vi "twoMPUsI2C.vi"() -> ()   [LabVIEW 2016]
uses:
  <vilib>/MakerHub/LINX/LMH-LINX.lvlib
  <vilib>/MakerHub/LINX/Public/Sensors/Accelerometer/MPU60X0/MPU60X0.lvlib
  <vilib>/MakerHub/LINX/Public/Sensors/Accelerometer/MPU60X0/AccelFullScaleRanges.ctl
  <vilib>/MakerHub/LINX/Public/Sensors/Accelerometer/MPU60X0/GyroFullScaleRanges.ctl
  <vilib>/MakerHub/LINX/Public/Initialize.vi
  <vilib>/MakerHub/LINX/Private/Type Defs/User Platform.ctl
  <vilib>/MakerHub/LINX/Public/Sensors/Accelerometer/MPU60X0/DeviceAddresses.ctl
  <vilib>/Platform/NI_3dgraph.lvlib
  <vilib>/MakerHub/LINX/Private/Type Defs/Interface.ctl
  <vilib>/MakerHub/LINX/Public/Sensors/Accelerometer/MPU60X0/Clock Source.ctl
panel:
  out "kthulu Chart":T1(graph)
  out "Path Length":dbl
  in  "I2C Channel":u8
  out "vector error":errorcluster
  in  "Plot of roll and pitch":refnum<k7>(container)
  out "XY Graph":cluster{"Y":dbl[], "Y":dbl[]}[](graph)
  out "error out":errorcluster
  out "MATLAB Error":errorcluster
  out "Error Out":errorcluster
  in  "?":bool
  in  "Clock Source":T2
  in  "Interface":T3
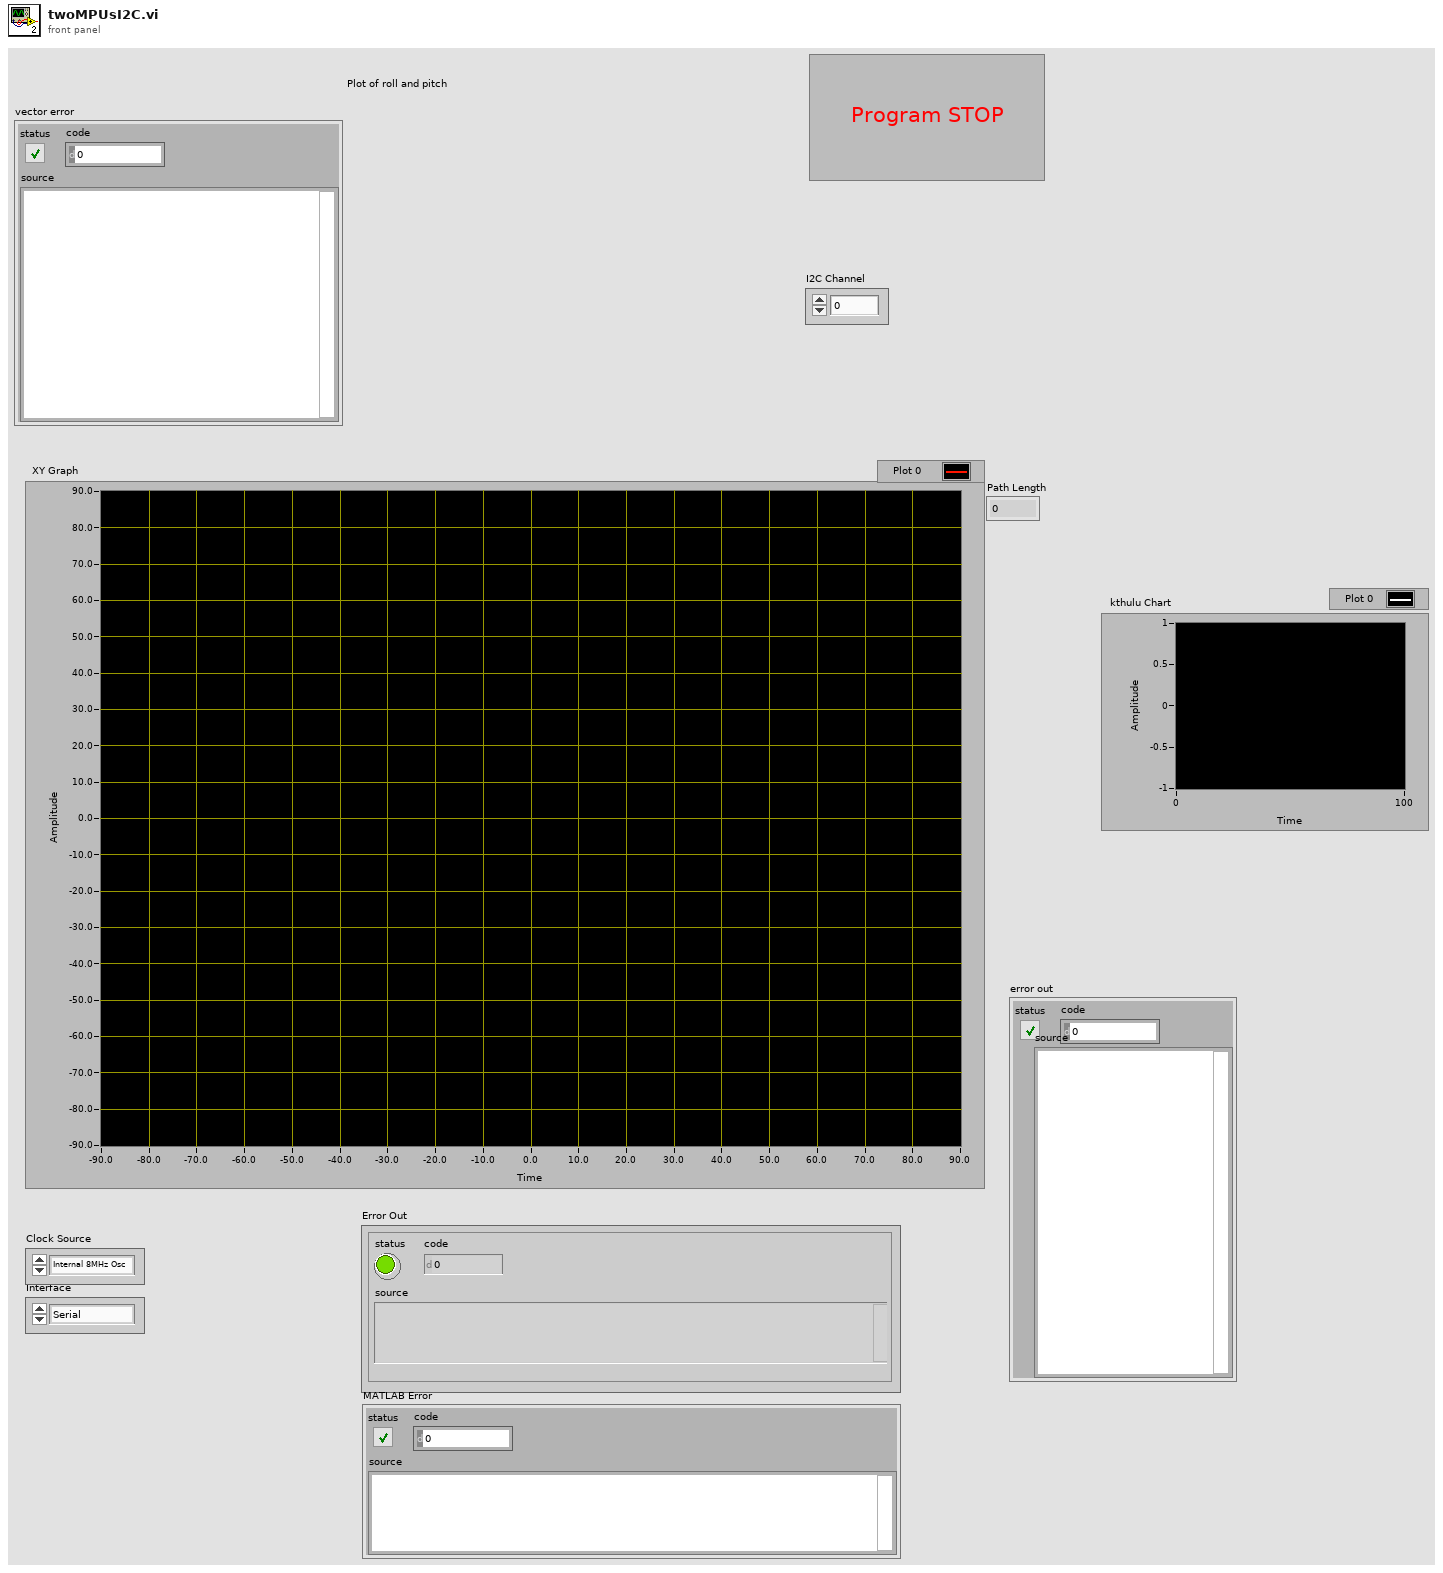
[diagram p1: front panel]
types:
  T1 = cluster{"X Axis":i16, "Y Axis":i16, "Z Axis":i16}
  T2 = typedef "LMH-LINX.lvlib/MPU60X0.lvlib/Clock Source.ctl" = enum8{"Internal 8MHz Osc", "PLL with X Gyro Ref", "PLL with Y Gyro Ref", "PLL with Z Gyro Ref", "PLL with ext 32.768 KHz Ref", "PLL with ext 19.2 MHz Ref", "Reserved", "Hold in reset"}
  T3 = typedef "LMH-LINX.lvlib/Interface.ctl" = enum16{"Serial", "TCP"}
  T4 = typedef "LMH-LINX.lvlib/MPU60X0.lvlib/DeviceAddresses.ctl" = enum16{"0x68", "0x69"}
  T5 = typedef "LMH-LINX.lvlib/MPU60X0.lvlib/GyroFullScaleRanges.ctl" = enum8{"±250 °/s", "±500 °/s", "±1000 °/s", "±2000 °/s"}
  T6 = typedef "LMH-LINX.lvlib/MPU60X0.lvlib/AccelFullScaleRanges.ctl" = enum16{"±2g", "±4g", "±8g", "±16g"}
  T7 = typedef "LMH-LINX.lvlib/User Platform.ctl" = enum16{"Default", "Remote", "Local"}
  T8 = typedef "LMH-LINX.lvlib/LINX Ref.ctl" = cluster{"IO":T9, "Interface":T3, "LINX Device Config":T10}
  T9 = typedef "LMH-LINX.lvlib/Platform.ctl" = enum16{"Remote", "Local"}
  T10 = typedef "LMH-LINX.lvlib/Device.lvlib/LINX Device Config.ctl" = cluster{"Interface":T3, "COM Port":refnum<visa-resource-name>, "TCP Configuration":T11, "Device Family":u8, "Device ID":u8, "Device Name":string, "TCP Ref":refnum<k5>, "Channels":T12}
  T11 = typedef "LMH-LINX.lvlib/Device.lvlib/TCP Config.ctl" = cluster{"IP Address":string, "Port":u16}
  T12 = typedef "LMH-LINX.lvlib/Channels.ctl" = cluster{"DI":u8[], "DO":u8[], "AI":u8[], "AO":u8[], "PWM":u8[], "QE":u8[], "UART":u8[], "I2C 2":u8[], "SPI":u8[], "CAN":u8[], "Servo":u8[], "AI Ref (V)":dbl, "AI Resolution (Bits)":u8, "AO Ref (V)":dbl, "AO Resolution (Bits)":u8}
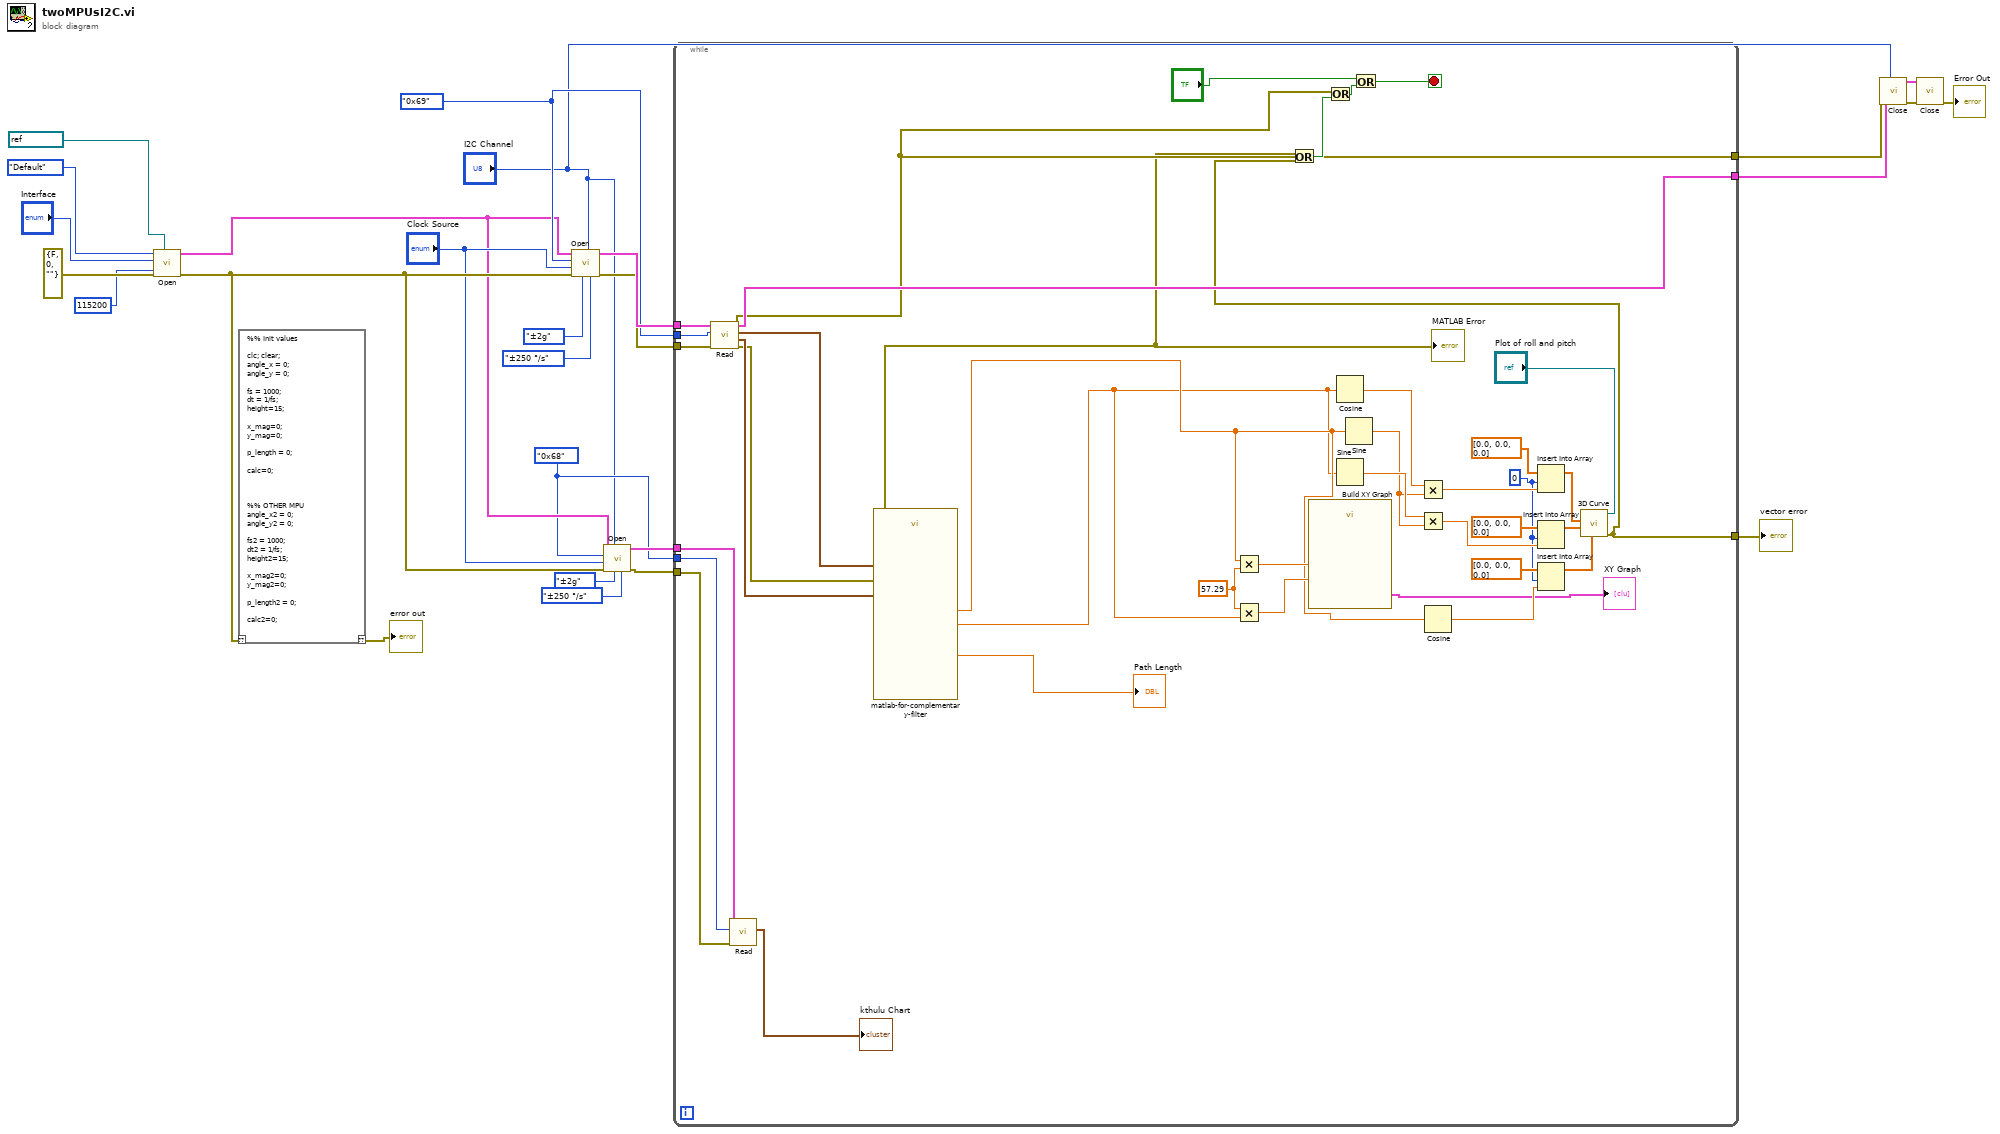
[diagram p0: block diagram]
diagram:
  w3 = DeviceAddresses."0x68" ("I2C Slave Address")
  w19 = DeviceAddresses."0x69" ("Device Address")
  n1 = call-poly <vilib>:"Open.vi"("Baud Rate Override"=u32 115200, "Serial Port"=refnum<visa-resource-name> "COM3", "Error In"=errorcluster {"status"=FALSE, "code"=0, "source"=""}, "Interface"="Interface", "IO"=User_Platform."Default") -> ("Error Out"=w7:errorcluster, "LINX Resource"=w5:T8)  [unwired: 4 in, 1 out]
  n2 = script code="%% Init values\n\nclc; clear;\nangle_x = 0;\nangle_y = 0;\n\nfs = 1000;\ndt = 1/fs;\nheight=15;\n\nx_mag=0; \ny_mag=0; \n\np_length = 0;\n\ncalc=0;\n\n\n\n%% OTHER MPU\nangle_x2 = 0;\nangle_y2 = 0;\n\nfs2 = 1000;\ndt2 = 1/fs;\nheight2=15;\n\nx_mag2=0; \ny_mag2=0; \n\np_length2 = 0;\n\ncalc2=0;"("??"=w7) -> ("??"=→"error out":errorcluster)
  n3 = call <vilib>:"Open.vi"("Gyro Full Scale Range"=GyroFullScaleRanges."±250 °/s", "Accel Full Scale Range"=AccelFullScaleRanges."±2g", "I2C Channel"="I2C Channel", "Error In"=w7, "Clock Source"="Clock Source", "I2C Slave Address"=w19, "LINX Resource"=w5) -> ("Error Out"=w20:errorcluster, "LINX Resource"=w21:T8)  [unwired: 3 in]
  n4 = call <vilib>:"Open.vi"("Gyro Full Scale Range"=GyroFullScaleRanges."±250 °/s", "Accel Full Scale Range"=AccelFullScaleRanges."±2g", "I2C Channel"="I2C Channel", "Error In"=w7, "Clock Source"="Clock Source", "I2C Slave Address"=w3, "LINX Resource"=w5) -> ("Error Out"=w2:errorcluster, "LINX Resource"=w4:T8)  [unwired: 3 in]
  n5 = while {
    tunnel: w21 -> [w65]
    tunnel: w20 -> [w64]
    tunnel: w19 -> [w63]
    tunnel: [w62] -> w18
    tunnel: [w33] -> w16
    tunnel: [w44] -> w10
    tunnel: w4 -> [w38]
    tunnel: w3 -> [w37]
    tunnel: w2 -> [w36]
    stop <- w46 stop-if-true
    w49 = 57.29 ("y")
    w50 = 0 ("index")
    n6 = call <vilib>:"Read.vi"("Error In"=w64, "I2C Slave Address"=w63, "LINX Resource"=w65) -> ("Error Out"=w33:errorcluster, "Gyro  Data (dps)"=w35:T1, "Acceleration Data (g)"=w34:T1, "LINX Resource"=w62:T8)  [unwired: 4 in, 1 out]
    n7 = call <vilib>:"Read.vi"("Error In"=w36, "I2C Slave Address"=w37, "LINX Resource"=w38) -> ("Acceleration Data (g)"=→"kthulu Chart":T1, "LINX Resource"=w27:T8)  [unwired: 4 in, 3 out]
    n8 = call "matlab-for-complementary-filter.vi"("Acceleration Data (g)"=w34, "Gyro  Data (dps)"=w35, "error in (no error)"=w33) -> ("angle_y"=w29:dbl, "Path Length"=→"Path Length":dbl, "angle_x"=w30:dbl, "error out"=w32:errorcluster)  [unwired: 11 in, 2 out]
    "MATLAB Error" <- w32
    n9 = Multiply(x=w30, y=w49) -> (x*y=w40:dbl)
    n10 = Multiply(x=w49, y=w29) -> (x*y=w39:dbl)
    n11 = call "Build XY Graph"("Y Input"=w39, "X Input"=w40) -> ("XY Graph"=→"XY Graph":cluster{"X":dbl[], "Y":dbl[]}[])  [unwired: 8 in, 1 out]
    n12 = Cosine(x=w29) -> (cos(x)=w61:dbl)
    n13 = Sine(x=w29) -> (sin(x)=w56:dbl)
    n14 = Sine(x=w30) -> (sin(x)=w55:dbl)
    n15 = Multiply(x=w61, y=w55) -> (x*y=w58:dbl)
    n16 = Multiply(x=w56, y=w55) -> (x*y=w54:dbl)
    n17 = Cosine(x=w30) -> (cos(x)=w52:dbl)
    n18 = Insert Into Array(array=dbl[] [0.0, 0.0, 0.0], index=w50, new element=w58) -> (w48:dbl[])
    n19 = Insert Into Array(array=dbl[] [0.0, 0.0, 0.0], index=w50, new element=w54) -> (w47:dbl[])
    n20 = Insert Into Array(array=dbl[] [0.0, 0.0, 0.0], index=w50, new element=w52) -> (w51:dbl[])
    n21 = call <vilib>:"3D Curve.vi"("z vector"=w51, "y vector"=w47, "x vector"=w48, "3D graph"="Plot of roll and pitch") -> ("error out"=w44:errorcluster)  [unwired: 6 in, 1 out]
    n22 = Or(x=w32, y=w44) -> (x .or. y?=w45:bool)
    n23 = Or(x=w33, y=w45) -> (x .or. y?=w42:bool)
    n24 = Or(x="?", y=w42) -> (x .or. y?=w46:bool)
  }
  "vector error" <- w10
  n25 = call <vilib>:"Close.vi"("I2C Channel (0)"="I2C Channel", "Error In"=w16, "LINX Resource"=w18) -> ("Error Out"=w15:errorcluster, "LINX Resource"=w17:T8)  [unwired: 7 in]
  n26 = call <vilib>:"Close.vi"("Error In"=w15, "LINX Resource"=w17) -> ("Error Out"=→"Error Out":errorcluster)  [unwired: 9 in]
